vi "15 Triple Phase Signal Generation (x64-2018).vi"(8 "Error In":errorcluster, 9 "Rate":dbl=1000.0, 10 "Number of samples per channel":dbl=40.0, 11 "task/channels in":refnum<k21>) -> (0 "Error Out":errorcluster, 2 "data":waveform(dbl)[](array[waveform]), 3 "task out":refnum<k21>)   [LabVIEW 2017]
uses:
  <vilib>/DAQmx/read.llb/DAQmx Read (Analog 1D Wfm NChan NSamp Duration).vi
  <vilib>/DAQmx/create/channels.llb/DAQmx Create Channel (AI-Voltage-Basic).vi
  <vilib>/DAQmx/configure/timing.llb/DAQmx Timing (Sample Clock).vi
  <vilib>/DAQmx/miscellaneous.llb/DAQmx Fill In Error Info.vi
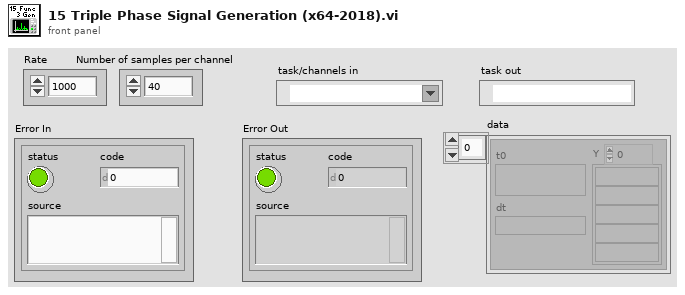
[diagram p1: front panel]
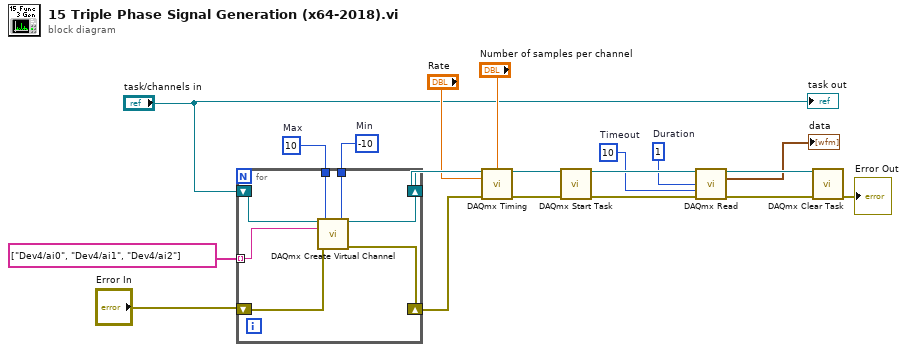
[diagram p0: block diagram]
diagram:
  w14 = 1  # Duration
  w15 = 10  # Timeout
  w19 = 10  # Max
  w18 = -10  # Min
  n1 = for {
    tunnel: w19 -> [w26]
    tunnel: w18 -> [w25]
    shift-right: [w23] -> w11
    shift-left: "Error In" -> [w22]
    shift-right: [w24] -> w13
    shift-left: "task/channels in" -> [w21]
    tunnel: string[] ["Dev4/ai0", "Dev4/ai1", "Dev4/ai2"] -> [w20] mode=indexing
    n2 = call-poly <vilib>:"DAQmx Create Virtual Channel.vi"("task in"=w21, "maximum value"=w26, "minimum value"=w25, "physical channels"=w20, "error in"=w22) -> ("task out"=w24:refnum<k21>, "error out"=w23:errorcluster)  [unwired: 9 in]
  }
  n3 = call-poly <vilib>:"DAQmx Timing.vi"("task/channels in"=w13, "samples per channel"="Number of samples per channel", "rate"="Rate", "error in"=w11) -> ("task out"=w12:refnum<k21>, "error out"=w10:errorcluster)  [unwired: 10 in]
  n4 = call <vilib>:"DAQmx Start Task.vi"("task/channels in"=w12, "error in"=w10) -> ("task out"=w17:refnum<k21>, "error out"=w16:errorcluster)  [unwired: 12 in]
  n5 = call-poly <vilib>:"DAQmx Read.vi"("task/channels in"=w17, "duration"=w14, "timeout"=w15, "error in"=w16) -> ("task out"=w9:refnum<k21>, "data"=→"data":waveform(dbl)[], "error out"=w8:errorcluster)  [unwired: 9 in]
  n6 = call <vilib>:"DAQmx Clear Task.vi"("task in"=w9, "error in"=w8) -> ("error out"=→"Error Out":errorcluster)  [unwired: 13 in]
  "task out" <- "task/channels in"
